vi "Log Data.vi"(8 "error in (no error)":errorcluster, 10 "Data Queue":refnum<queue>, 11 "Logging Configuration":T1) -> (0 "error out":errorcluster)   [LabVIEW 2016, in "Logging.lvlib"]
doc: "This VI uses the TDMS Write function to write data to a TDMS file."
uses:
  Logging.lvlib
  Logging Configuration.ctl
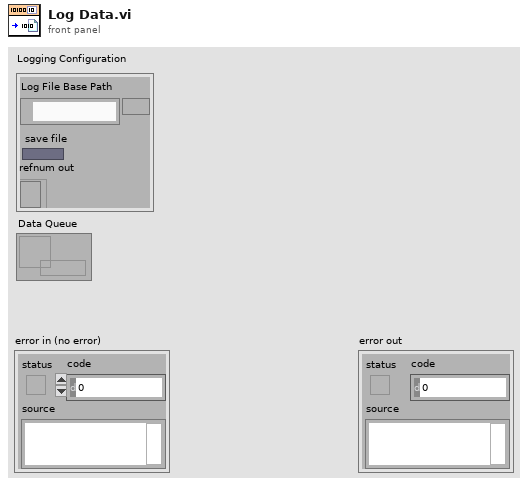
[diagram p1: front panel]
types:
  T1 = typedef "Logging.lvlib/Logging Configuration.ctl" = cluster{"Log File Base Path":path, "save file":bool, "refnum out":refnum<file>}
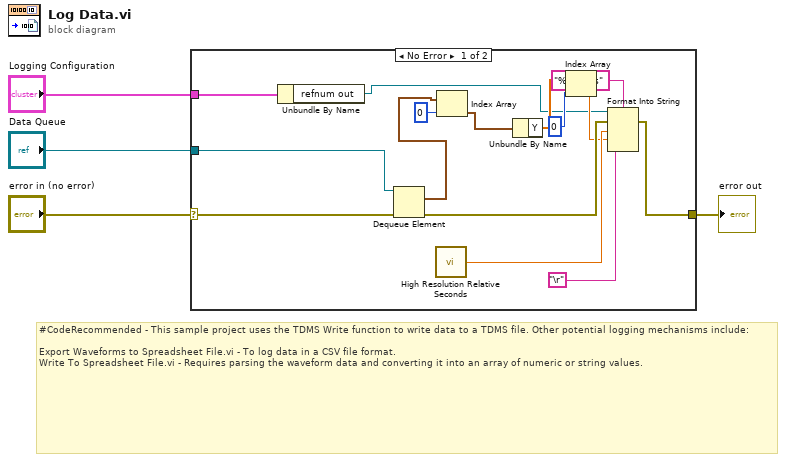
[diagram p0: block diagram]
diagram:
  # "#CodeRecommended - This sample project uses the TDMS Write function to write data to a TDMS file. Other potential logging mechanisms include:\n\nExport Waveforms to Spreadsheet File.vi - To log data in a CSV file format.\nWrite To Spreadsheet File.vi - Requires parsing the waveform data and converting it into an array of numeric or string values."
  n1 = case shown="No Error" "error in (no error)" {
    selector: "error in (no error)" -> [w18 w20]
    tunnel: "Logging Configuration" -> [w19 _]
    tunnel: "Data Queue" -> [w17 _]
    tunnel: [w15 w20] -> w2
    frame No Error {
      n2 = Unbundle By Name(w19) -> ("refnum out"=w5:refnum<file>)
      n3 = Dequeue Element(queue=w17, error in (no error)=w18) -> (element=w10:waveform(dbl)[], error out=w16:errorcluster)  [unwired: 1 in, 2 out]
      n4 = call <vilib>:"High Resolution Relative Seconds.vi"() -> ("relative seconds"=w9:dbl)
      n5 = Index Array(array=w10, index=0) -> (element=w13:waveform(dbl))
      n6 = Unbundle By Name(w13) -> ("Y"=w12:dbl[])
      n7 = Index Array(array=w12, index=0) -> (element=w8:dbl)
      n8 = Format Into String(format string="%f,%f%s", initial string=w5, error in=w16, w9, w8, "\r") -> (error out=w15:errorcluster)  [unwired: 1 out]
    }
    frame Error {
    }
  }
  "error out" <- w2
